vi "Calculate single run.vi"(7 "Position":refnum<class "Position.lvclass">, 8 "error in (no error)":errorcluster, 9 "Direction":T1, 10 "Source":T2={"File"=enum."d", "Rank"=enum."4"}) -> (0 "error out":errorcluster, 2 "Destinations":T2[](array[typedef]))   [LabVIEW 2016, in "Chesslib.lvlib" / "Runner.lvclass"]
uses:
  Runner.lvclass
  Position/Position.lvclass
  typedef/Square.ctl
  typedef/File.ctl
  typedef/Rank.ctl
  typedef/Neighbor.ctl
  Chesslib.lvlib
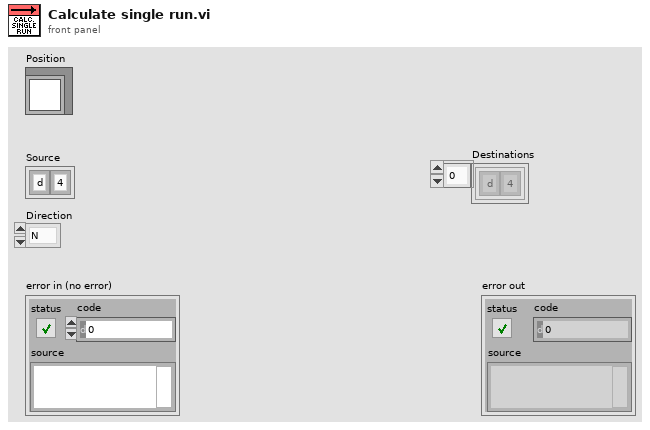
[diagram p1: front panel]
types:
  T1 = typedef "Chesslib.lvlib/Neighbor.ctl" = enum16{"N", "NW", "W", "SW", "S", "SE", "E", "NE", "vector"}
  T2 = typedef "Chesslib.lvlib/Square.ctl" = cluster{"File":T3, "Rank":T4}
  T3 = typedef "Chesslib.lvlib/File.ctl" = enum8{"a", "b", "c", "d", "e", "f", "g", "h"}
  T4 = typedef "Chesslib.lvlib/Rank.ctl" = enum8{"1", "2", "3", "4", "5", "6", "7", "8"}
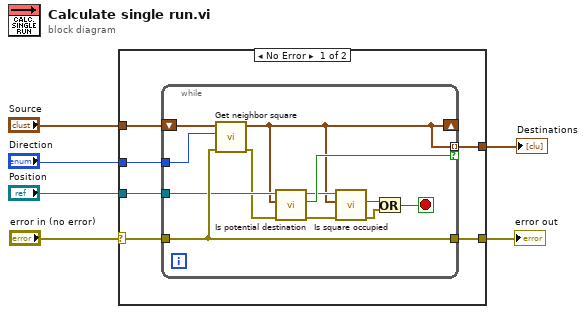
[diagram p0: block diagram]
diagram:
  n1 = case shown="No Error" "error in (no error)" {
    selector: "error in (no error)" -> [w8 w25]
    tunnel: "Source" -> [w12 _]
    tunnel: "Position" -> [w11 _]
    tunnel: [w10 _] -> w4
    tunnel: "Direction" -> [w9 _]
    tunnel: [w7 w25] -> w1
    frame No Error {
      n2 = while {
        tunnel: w9 -> [w24]
        tunnel: w11 -> [w21]
        shift-right: [w13] -> _
        shift-left: w12 -> [w23]
        tunnel: [w13] -> w10 mode=indexing if=w20
        tunnel: w8 -> [w22]
        tunnel: [w22] -> w7
        stop <- w17 stop-if-true
        n3 = call "Get neighbor square.vi"("error in (no error)"=w22, "Neighbor (vector)"=w24, "Square in"=w23) -> ("error out"=w16:errorcluster, "Square out"=w13:T2)  [unwired: 6 in, 1 out]
        n4 = call "Is potential destination.vi"("error in (no error)"=w16, "Square"=w13, "Position in"=w21) -> ("error out"=w15:errorcluster, "Potential destination"=w20:bool, "Position out"=w19:refnum<class "Position.lvclass">)  [unwired: 6 in]
        n5 = call "Is square occupied.vi"("error in (no error)"=w15, "Square"=w13, "Position in"=w19) -> ("error out"=w14:errorcluster, "Occupied"=w18:bool)  [unwired: 6 in, 1 out]
        n6 = Or(x=w18, y=w14) -> (x .or. y?=w17:bool)
      }
    }
    frame Error {
    }
  }
  "Destinations" <- w4
  "error out" <- w1
